vi "sub_file-path.vi"(7 "cmd":enum16{"create", "save"}(ring), 8 "error in (no error)":errorcluster caption="에러 입력(에러 없음)", 11 "data":string) -> (0 "error out":errorcluster caption="에러 출력")   [LabVIEW 2013]
panel:
  out "appended path":path
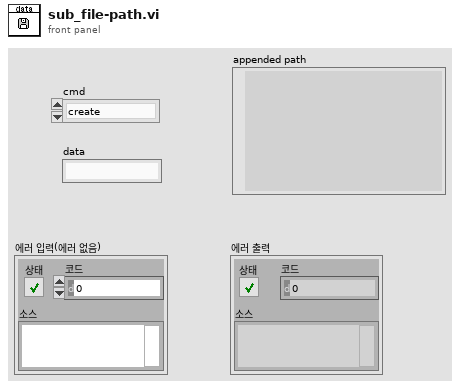
[diagram p1: front panel]
types:
  T1 = enum16{"open", "replace", "create", "open or create", "replace or create", "replace or create with confirmation"}
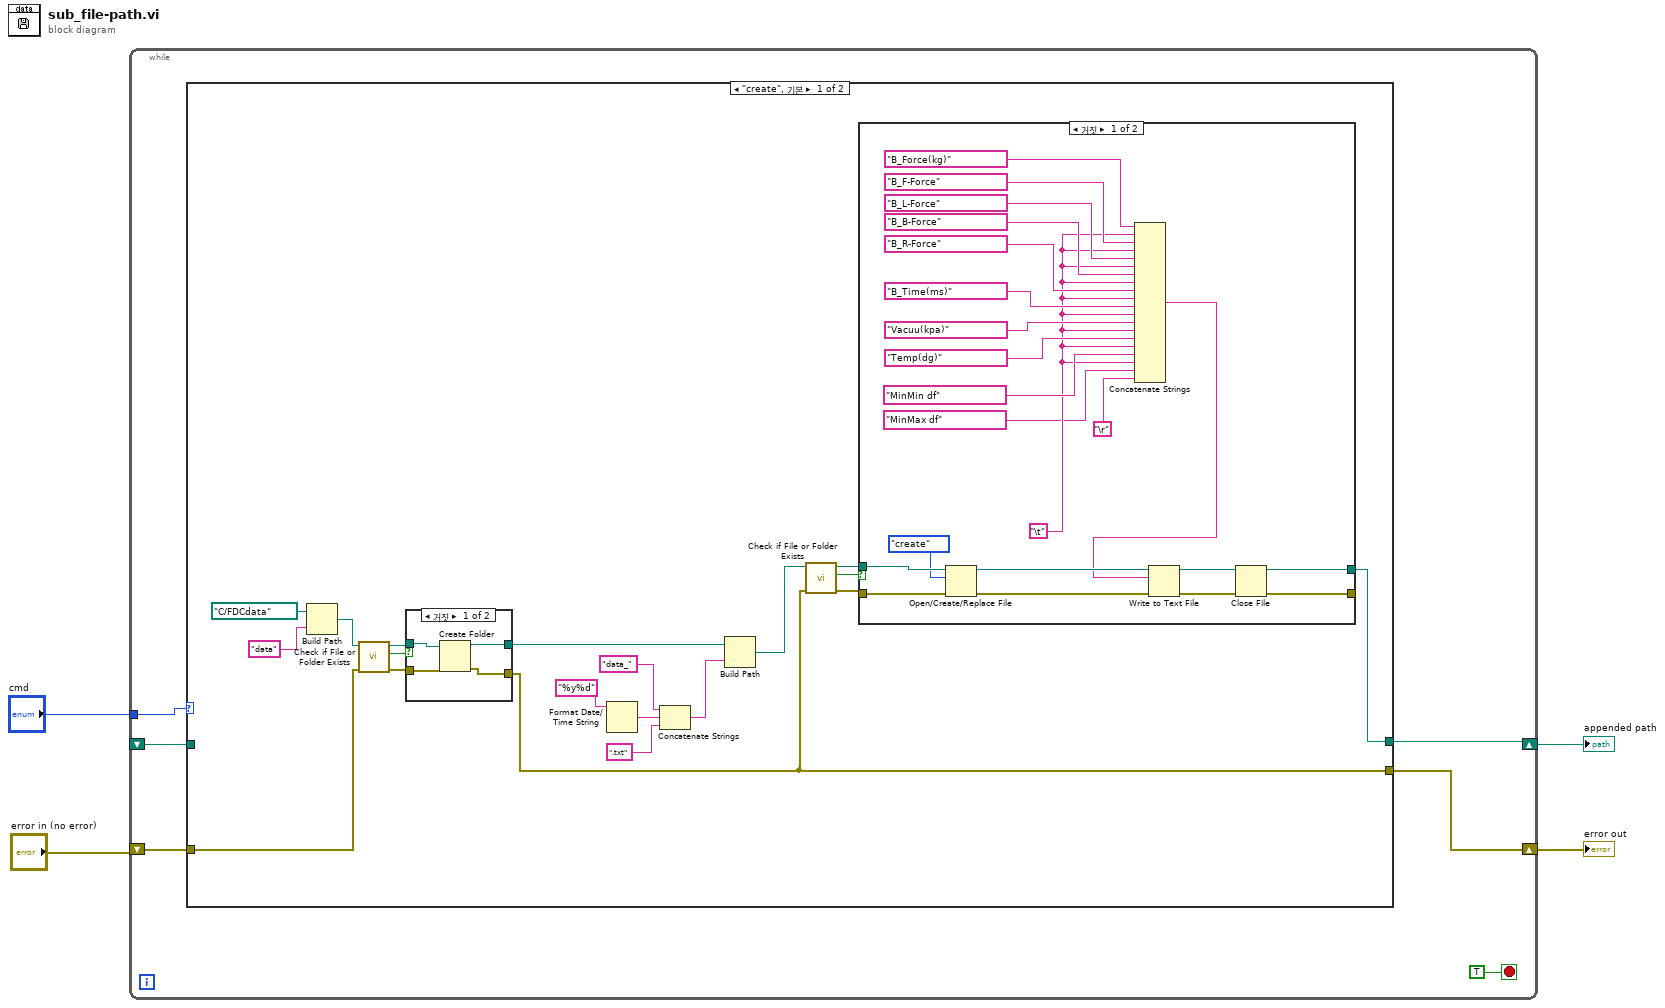
[diagram p0: block diagram]
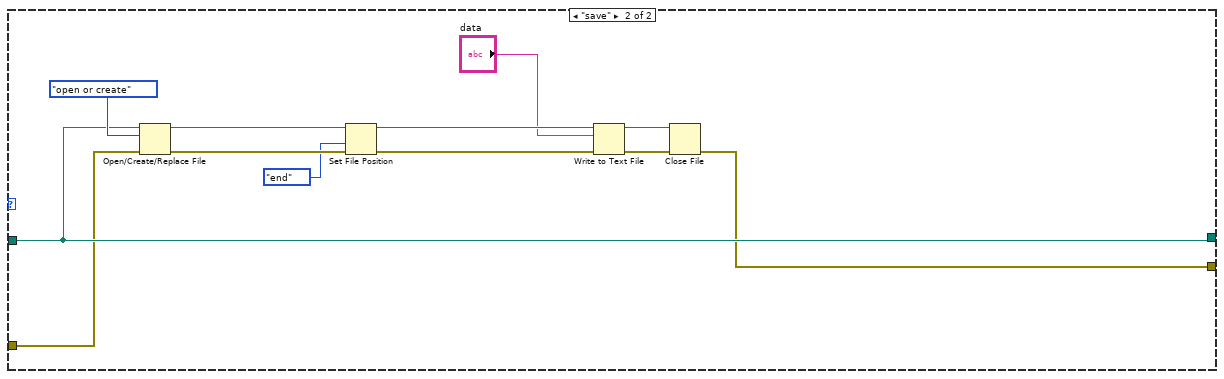
[diagram p4: hidden frame]
diagram:
  n1 = while {
    tunnel: "cmd" -> [w10]
    shift-right: [w7] -> w2
    shift-left: "error in (no error)" -> [w8]
    shift-right: [w6] -> w1
    shift-left: _ -> [w5]
    stop <- TRUE stop-if-true
    n2 = case shown="\"create\", 기본" w10 {
      tunnel: w8 -> [w22 w62]
      tunnel: [w15 w61] -> w7
      tunnel: [w14 w68] -> w6
      tunnel: w5 -> [_ w68]
      frame "create", Default {
        n3 = Build Path(base path=path "C:/FDCdata" ("베이스 경로"), name or relative path="data" ("이름 또는 상대 경로")) -> (appended path=w25:path)
        n4 = call <vilib>:"Check if File or Folder Exists.vi"("error in (no error)"=w22, "path"=w25) -> ("error out"=w29:errorcluster, "file or folder exists?"=w28:bool, "dup path"=w27:path)  [unwired: 7 in]
        n5 = case shown="거짓" w28 {
          tunnel: w27 -> [w57 w59]
          tunnel: w29 -> [w56 w58]
          tunnel: [w55 w59] -> w24
          tunnel: [w54 w58] -> w15
          frame False {
            n6 = Create Folder(path (use dialog)=w57, error in=w56) -> (created path=w55:path, error out=w54:errorcluster)  [unwired: 1 in, 1 out]
          }
          frame True {
          }
        }
        n7 = Format Date/Time String(time format string (%c)="%y%d" ("시간 포맷 문자열 (%c)")) -> (date/time string=w12:string)  [unwired: 2 in]
        n8 = Concatenate Strings("data_" ("이름 또는 상대 경로"), w12, ".txt" ("문자열")) -> (w20:string)
        n9 = Build Path(base path=w24, name or relative path=w20) -> (appended path=w19:path)
        n10 = call <vilib>:"Check if File or Folder Exists.vi"("error in (no error)"=w15, "path"=w19) -> ("error out"=w16:errorcluster, "file or folder exists?"=w18:bool, "dup path"=w17:path)  [unwired: 7 in]
        n11 = case shown="거짓" w18 {
          tunnel: w17 -> [w51 w52]
          tunnel: w16 -> [w50 w53]
          tunnel: [w44 w53] -> _
          tunnel: [w33 w52] -> w14
          frame False {
            w31 = "\t"
            n12 = Open/Create/Replace File(file path (use dialog)=w51, error in=w50, operation (0:open)=T1."create" ("동작(0:open)")) -> (refnum out=w47:refnum<file>, error out=w48:errorcluster)  [unwired: 3 in, 1 out]
            n13 = Concatenate Strings("B_Force(kg)", w31, "B_F-Force", w31, "B_L-Force", w31, "B_B-Force", w31, "B_R-Force", w31, "B_Time(ms)", w31, "Vacuu(kpa)", w31, "Temp(dg)", w31, "MinMin df", w31, "MinMax df", "\r") -> (w35:string)
            n14 = Write to Text File(file (use dialog)=w47, text=w35, error in=w48) -> (refnum out=w46:refnum<file>, error out=w45:errorcluster)  [unwired: 1 in, 1 out]
            n15 = Close File(refnum=w46, error in=w45) -> (path=w33:path, error out=w44:errorcluster)
          }
          frame True {
          }
        }
      }
      frame "save" {
        n16 = Open/Create/Replace File(file path (use dialog)=w68, error in=w62, operation (0:open)=T1."open or create" ("동작(0:open)")) -> (refnum out=w65:refnum<file>, error out=w67:errorcluster)  [unwired: 3 in, 1 out]
        n17 = Set File Position(refnum=w65, from (0:start)=enum16{"start", "end", "current"}."end" ("시작(0:시작)"), error in=w67) -> (refnum out=w64:refnum<file>, error out=w66:errorcluster)  [unwired: 1 in]
        n18 = Write to Text File(file (use dialog)=w64, text="data", error in=w66) -> (refnum out=w70:refnum<file>, error out=w71:errorcluster)  [unwired: 1 in, 1 out]
        n19 = Close File(refnum=w70, error in=w71) -> (error out=w61:errorcluster)  [unwired: 1 out]
      }
    }
  }
  "error out" <- w2
  "appended path" <- w1
